vi "Plotter_UI_Event_Handler.vi"(8 "error in (no error)":errorcluster, 11 "Globals":T1) -> (0 "error out":errorcluster)   [LabVIEW 2017]
uses:
  Controls/Plotter_Globals.ctl
  Classes/ADCP.lvclass
  Controls/Plotter_Queues.ctl
  Controls/Plotter_Queue_Command_and_Data.ctl
  Controls/Plotter_Commands.ctl
  Controls/Plotter_Parameter_List_Record.ctl
panel:
  out "Send parameter":bool
  out "Exit Application":bool
  out "Enable / disable node connection":bool
  out "Remove receive parameter":bool
  out "Add receive parameter":bool
  out "Set Session Name":bool
  out "Load Symbol File":bool
  out "Serial Port Connection":bool
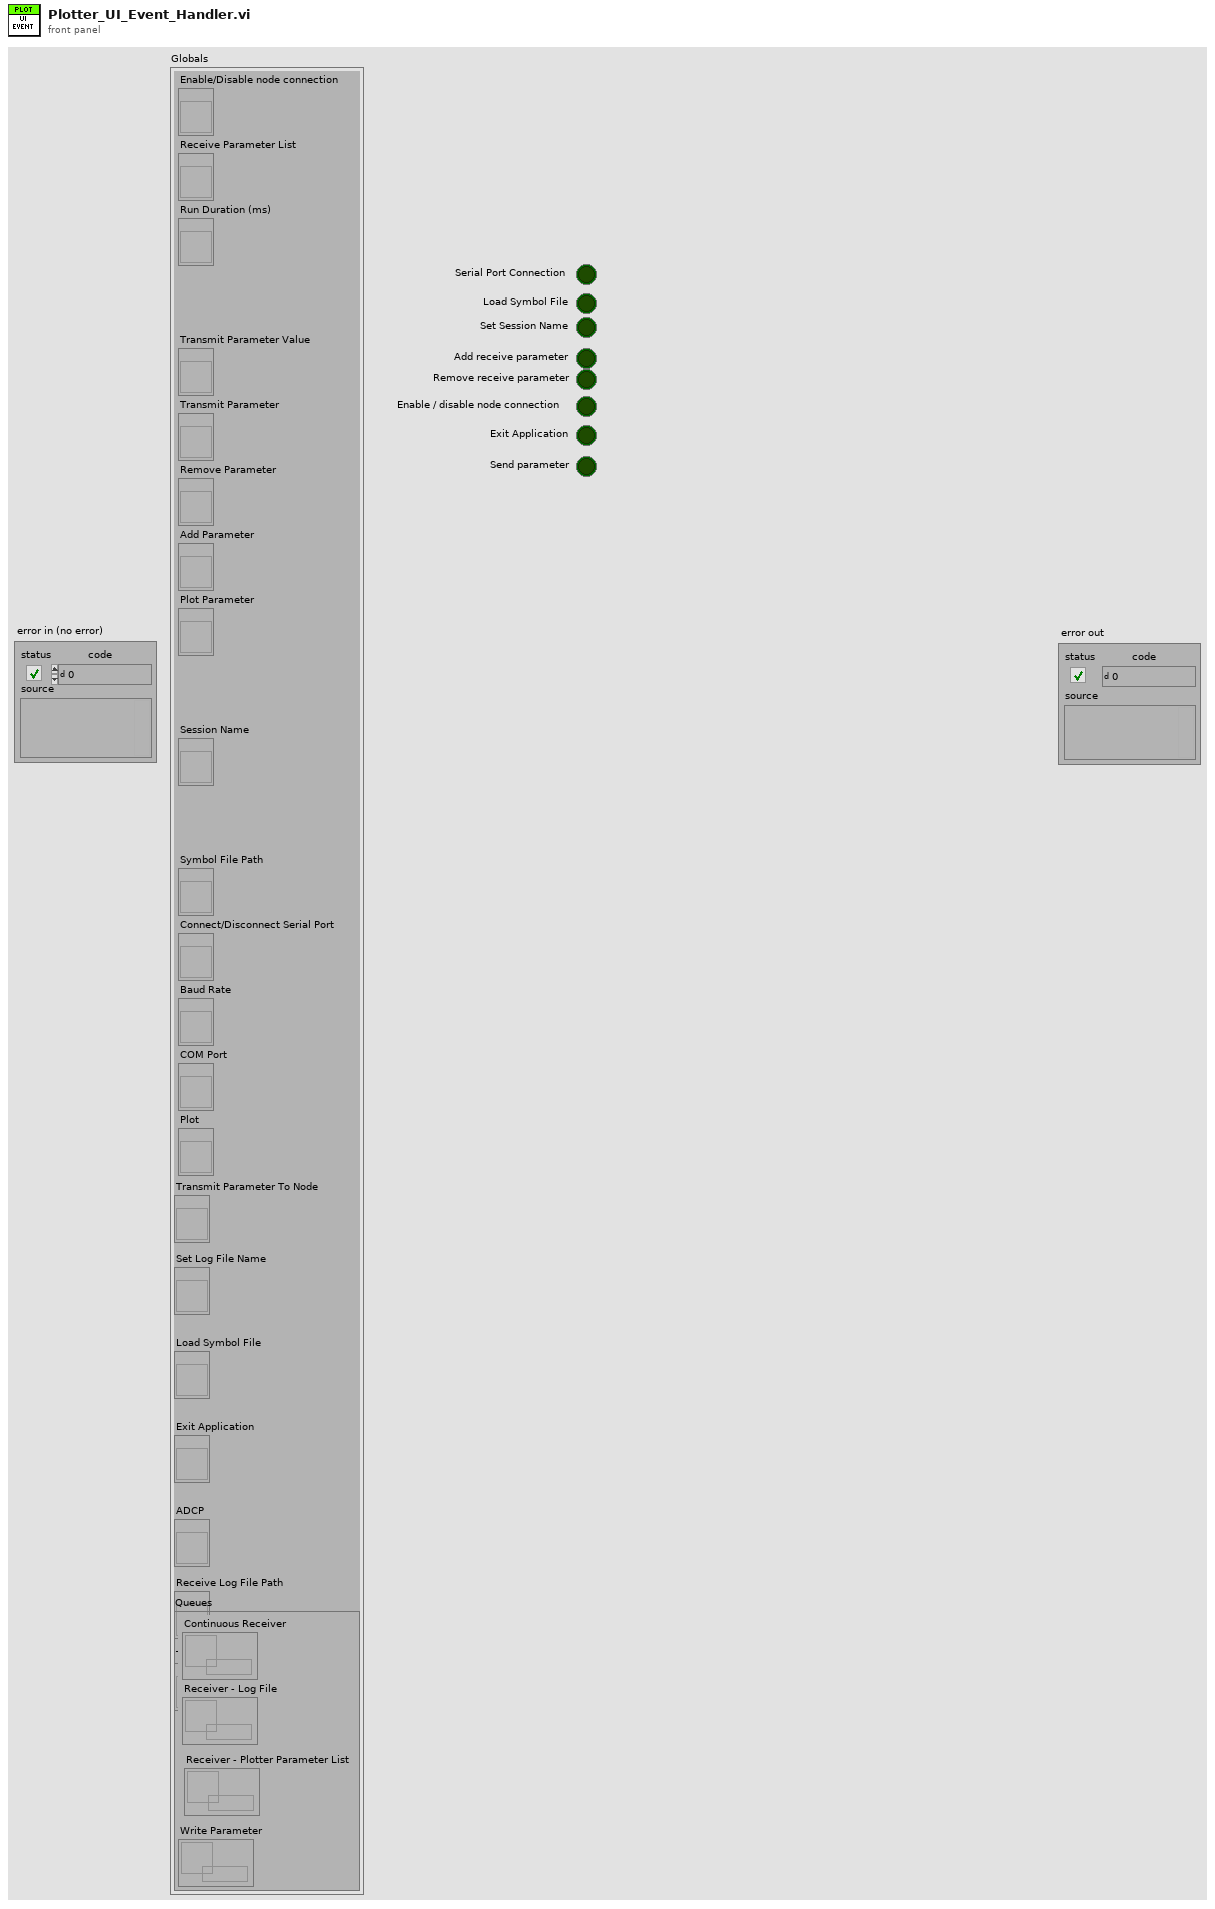
[diagram p1: front panel]
types:
  T1 = typedef "Plotter_Globals.ctl" = cluster{"Enable/Disable node connection":refnum<vi>, "Receive Parameter List":refnum<vi>, "Run Duration (ms)":refnum<vi>, "Transmit Parameter Value":refnum<vi>, "Transmit Parameter":refnum<vi>, "Remove Parameter":refnum<vi>, "Add Parameter":refnum<vi>, "Plot Parameter":refnum<vi>, "Session Name":refnum<vi>, "Symbol File Path":refnum<vi>, "Connect/Disconnect Serial Port":refnum<vi>, "Baud Rate":refnum<vi>, "COM Port":refnum<vi>, "Plot":refnum<vi>, "Transmit Parameter To Node":refnum<vi>, "Set Log File Name":refnum<vi>, "Load Symbol File":refnum<vi>, "Exit Application":refnum<vi>, "ADCP":refnum<vi>, "Transmit Log File Path":refnum<vi>, "Receive Log File Path":refnum<vi>, "Queues":T2}
  T2 = typedef "Plotter_Queues.ctl" = cluster{"Continuous Receiver":refnum<queue>, "Receiver - Log File":refnum<queue>, "Receiver - Plotter Parameter List":refnum<queue>, "Write Parameter":refnum<queue>}
  T3 = typedef "Plotter_Queue_Command_and_Data.ctl" = cluster{"Commands":T4, "Data":variant}
  T4 = typedef "Plotter_Commands.ctl" = enum16{"Idle", "Cont_RX_Open_Node", "Cont_RX_Flush_Serial_Port", "Cont_Rx_Log_Write", "Plot_Update", "Exit"}
  T5 = cluster{"Symbol File Path":path, "Transmit Log File Path":path, "Receive Log File Path":path, "COM Port":refnum<visa-resource-name>, "Baud rate":u32, "Number of retries":u16, "Retry interval (ms)":u16, "Session start time (ms)":u32, "Current time (ms)":u32, "Serialport timeout (ms)":u32}
  T6 = typedef "Plotter_Parameter_List_Record.ctl" = cluster{"Parameter":string, "Value":string}
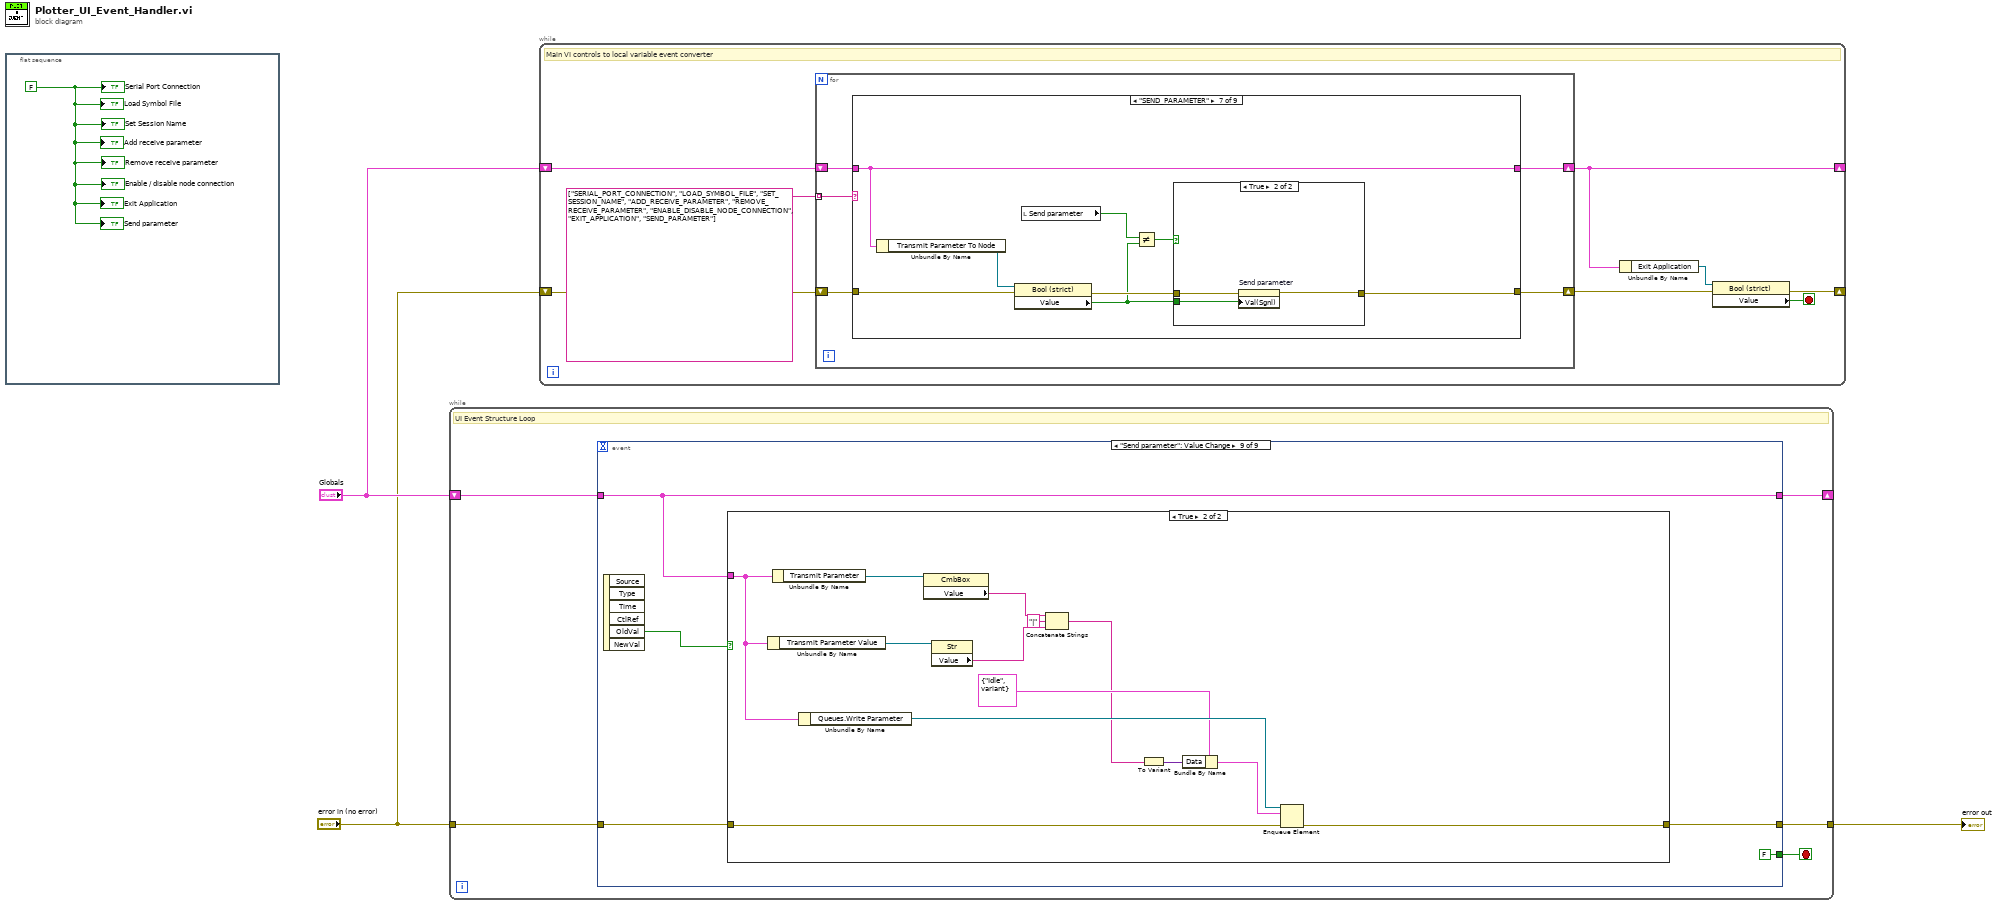
[diagram p0: block diagram]
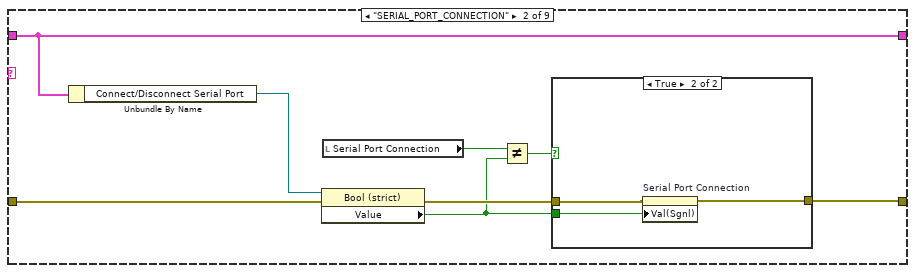
[diagram p3: hidden frame]
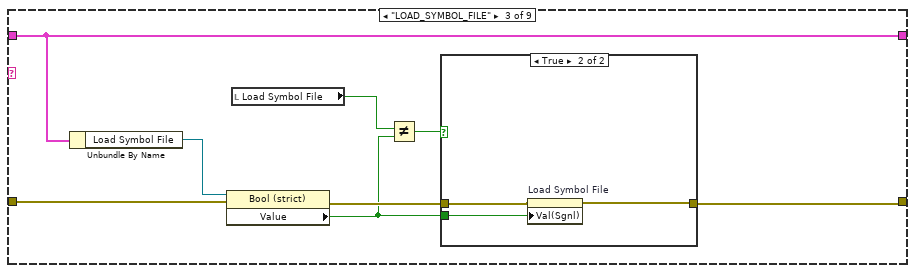
[diagram p5: hidden frame]
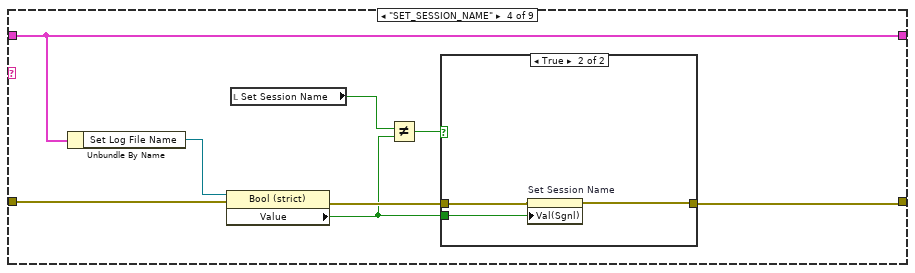
[diagram p7: hidden frame]
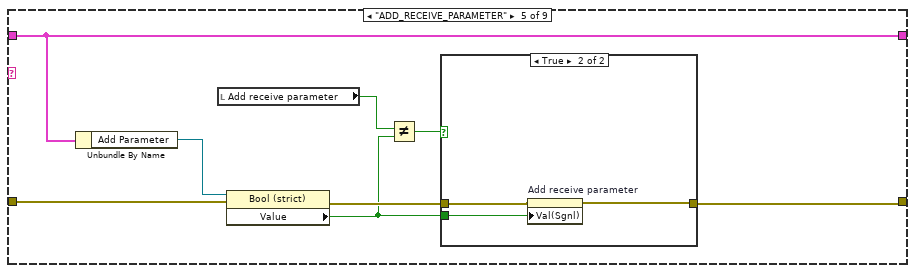
[diagram p9: hidden frame]
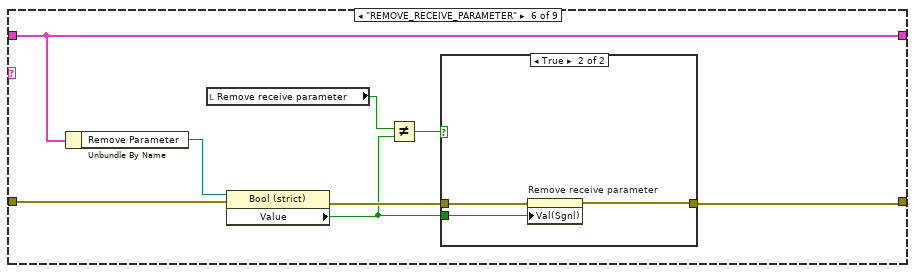
[diagram p11: hidden frame]
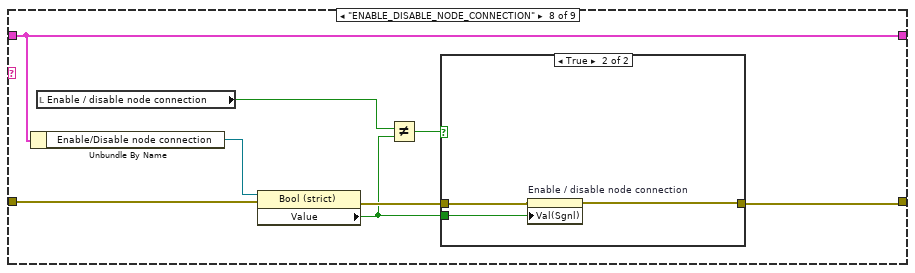
[diagram p14: hidden frame]
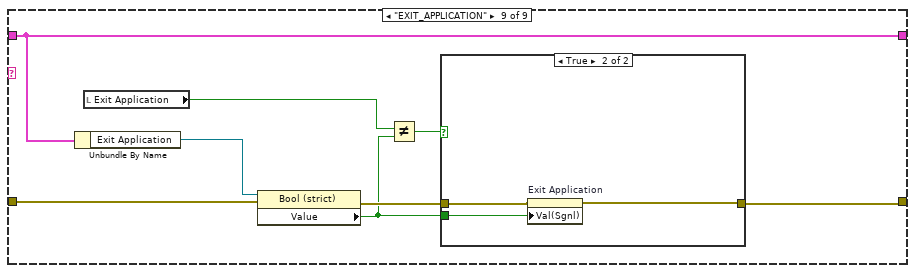
[diagram p16: hidden frame]
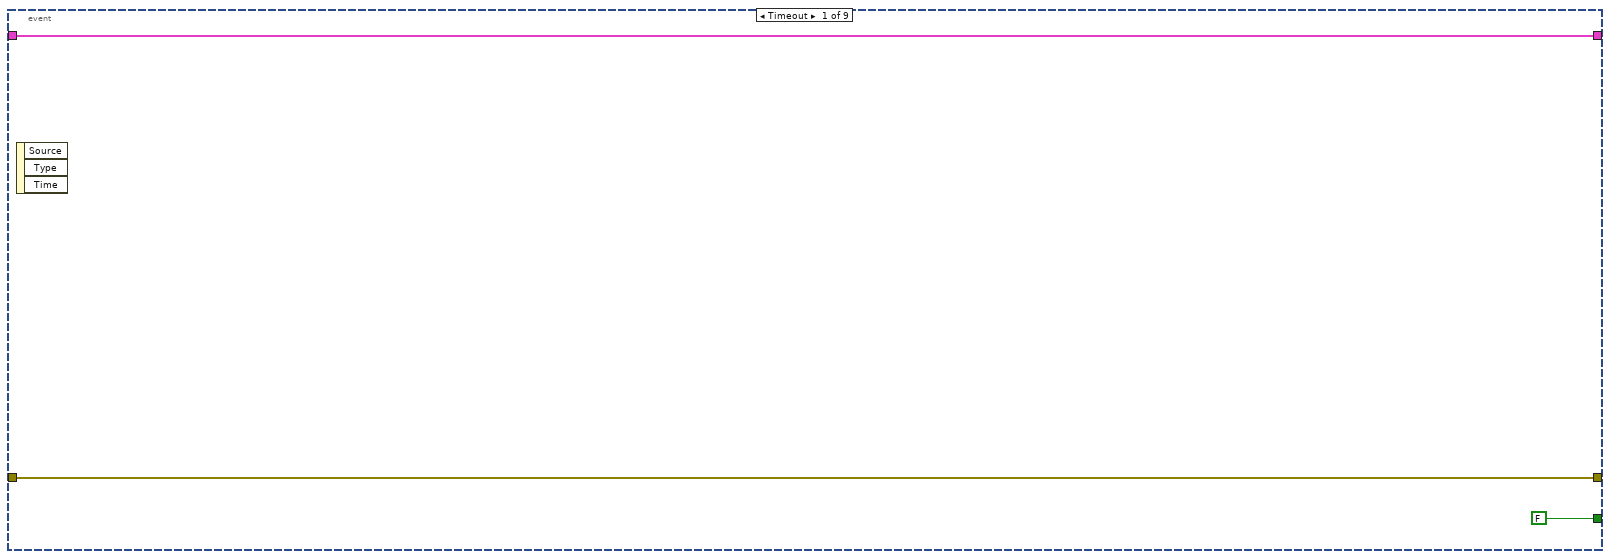
[diagram p18: hidden frame]
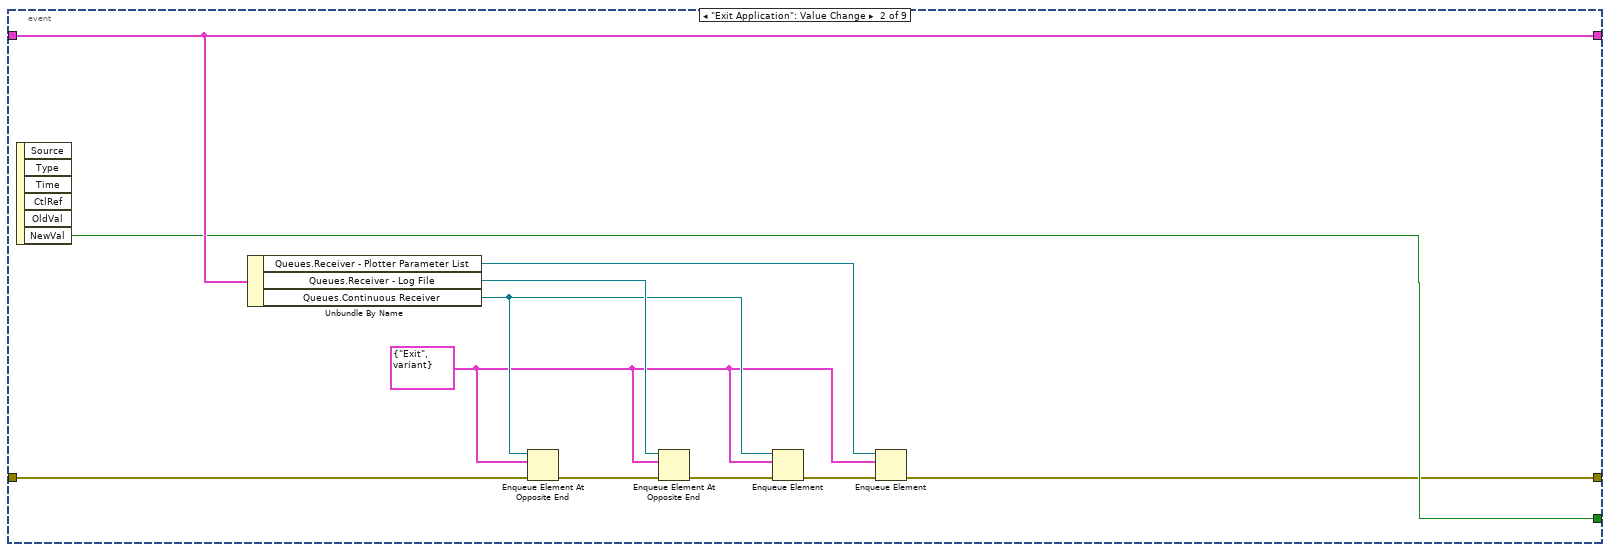
[diagram p19: hidden frame]
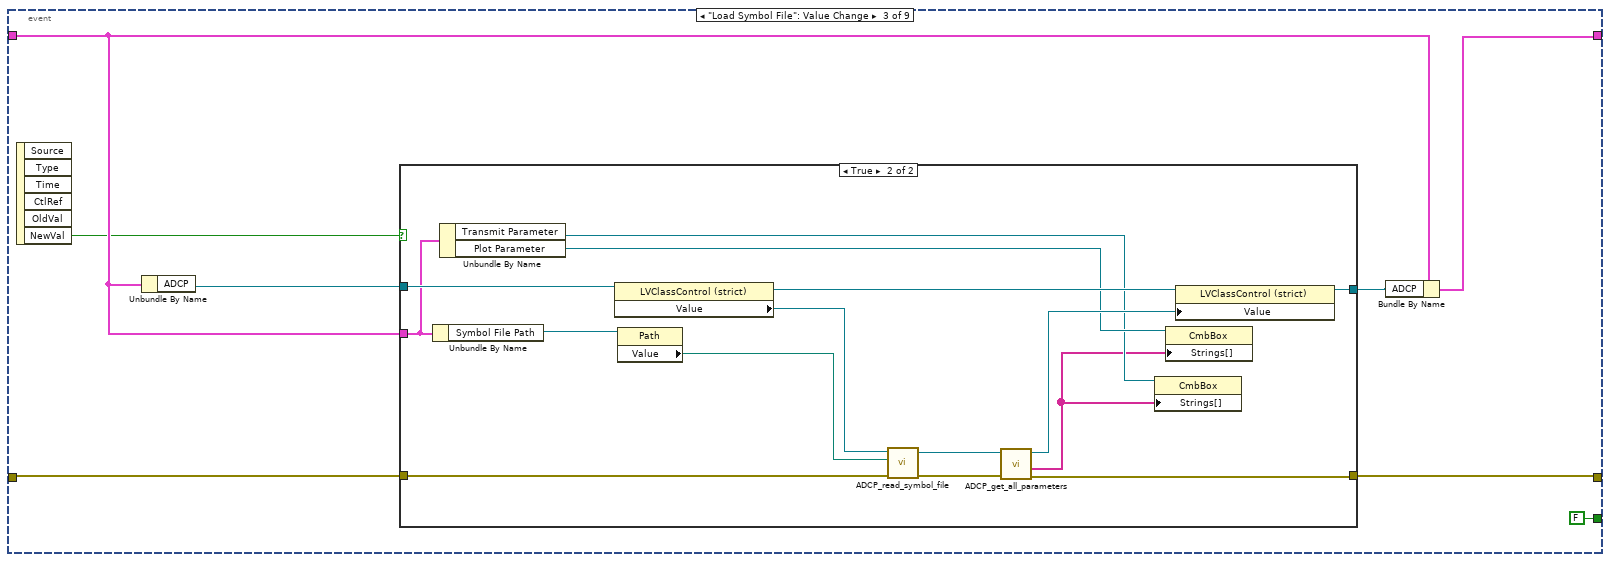
[diagram p20: hidden frame]
diagram:
  n1 = flat-sequence {
    frame #0 {
      w4 = FALSE ("Serial Port Connection")
      "Serial Port Connection" <- w4
      "Load Symbol File" <- w4
      "Set Session Name" <- w4
      "Add receive parameter" <- w4
      "Remove receive parameter" <- w4
      "Enable / disable node connection" <- w4
      "Exit Application" <- w4
      "Send parameter" <- w4
    }
  }
  n2 = while {
    shift-right: [w8] -> _
    shift-left: "Globals" -> [w9]
    tunnel: "error in (no error)" -> [w6]
    tunnel: [w5] -> w3
    stop <- w7 stop-if-true
    # "UI Event Structure Loop"
    n3 = event shown="[8] \"Send parameter\": Value Change" {
      selector: _ -> [_ _ _ _ _ _ _ _ _]
      dyn-events: _ -> [_ _ _ _ _ _ _ _ _]
      timeout: _ -> [_ _ _ _ _ _ _ _ _]
      tunnel: w9 -> [w12 w23 w27 w50 w68 w105 w130 w156 w175]
      tunnel: [w12 w23 w25 w49 w67 w103 w129 w155 w175] -> w8
      tunnel: [FALSE w17 FALSE FALSE FALSE FALSE FALSE ("NewVal") FALSE ("NewVal") FALSE ("NewVal")] -> w7
      tunnel: w6 -> [w10 w22 w31 w52 w69 w101 w131 w157 w177]
      tunnel: [w10 w15 w28 w51 w66 w100 w127 w153 w176] -> w5
      event Timeout {
        n4 = event-data() -> ()  [unwired: 1 in, 3 out]
      }
      event "Exit Application": Value Change {
        w13 = T3 {"Commands"=enum."Exit", "Data"=variant} ("element")
        n5 = event-data() -> ("NewVal"=w17:bool)  [unwired: 1 in, 5 out]
        n6 = Unbundle By Name(w23) -> ("Queues.Receiver - Plotter Parameter List"=w14:refnum<queue>, "Queues.Receiver - Log File"=w20:refnum<queue>, "Queues.Continuous Receiver"=w18:refnum<queue>)
        n7 = Enqueue Element At Opposite End(queue=w18, element=w13, error in (no error)=w22) -> (error out=w21:errorcluster)  [unwired: 1 in, 2 out]
        n8 = Enqueue Element At Opposite End(queue=w20, element=w13, error in (no error)=w21) -> (error out=w19:errorcluster)  [unwired: 1 in, 2 out]
        n9 = Enqueue Element(queue=w18, element=w13, error in (no error)=w19) -> (error out=w16:errorcluster)  [unwired: 1 in, 2 out]
        n10 = Enqueue Element(queue=w14, element=w13, error in (no error)=w16) -> (error out=w15:errorcluster)  [unwired: 1 in, 2 out]
      }
      event "Load Symbol File": Value Change {
        n11 = event-data() -> ("NewVal"=w24:bool)  [unwired: 1 in, 5 out]
        n12 = Unbundle By Name(w27) -> ("ADCP"=w30:refnum<vi>)
        n13 = case shown="True" w24 {
          tunnel: w31 -> [w32 w48]
          tunnel: w30 -> [w33 w47]
          tunnel: [w32 w40] -> w28
          tunnel: w27 -> [_ w37]
          tunnel: [w33 w42] -> w26
          frame False {
          }
          frame True {
            n14 = Unbundle By Name(w37) -> ("Symbol File Path"=w45:refnum<vi>)
            n15 = Unbundle By Name(w37) -> ("Transmit Parameter"=w35:refnum<vi>, "Plot Parameter"=w36:refnum<vi>)
            n16 = property class="LVClassControl (strict)"(reference=w47) -> (reference out=w43:refnum<vi>, "Value"=w46:refnum<class "ADCP.lvclass">)  [unwired: 1 in, 1 out]
            n17 = property class="Path"(reference=w45) -> ("Value"=w44:path)  [unwired: 1 in, 2 out]
            n18 = call "ADCP_read_symbol_file.vi"("error in (no error)"=w48, "Symbol File Path"=w44, "ADCP in"=w46) -> ("error out"=w41:errorcluster, "ADCP out"=w39:refnum<class "ADCP.lvclass">)  [unwired: 5 in, 2 out]
            n19 = call "ADCP_get_all_parameters.vi"("error in (no error)"=w41, "ADCP In"=w39) -> ("error out"=w40:errorcluster, "Parameter names"=w34:string[], "ADCP Out"=w38:refnum<class "ADCP.lvclass">)  [unwired: 6 in, 1 out]
            n20 = property class="CmbBox"(reference=w35, "Strings[]"=w34) -> ()  [unwired: 1 in, 2 out]
            n21 = property class="CmbBox"(reference=w36, "Strings[]"=w34) -> ()  [unwired: 1 in, 2 out]
            n22 = property class="LVClassControl (strict)"(reference=w43, "Value"=w38) -> (reference out=w42:refnum<vi>)  [unwired: 1 in, 1 out]
          }
        }
        n23 = Bundle By Name(cluster=w27, "ADCP"=w26) -> (w25:T1)
      }
      event "Set Session Name": Value Change {
        n24 = event-data() -> ("NewVal"=w53:bool)  [unwired: 1 in, 5 out]
        n25 = case shown="True" w53 {
          tunnel: w52 -> [w56 w64]
          tunnel: [w56 w60] -> w51
          tunnel: w50 -> [w55 w59]
          tunnel: [w55 w59] -> w49
          frame False {
          }
          frame True {
            n26 = Unbundle By Name(w59) -> ("Session Name"=w58:refnum<vi>)
            n27 = property class="Str"(reference=w58) -> ("Value"=w57:string)  [unwired: 1 in, 2 out]
            n28 = call "Transmit_Log_File_FGV.vi"("Session name"=w57, "error in (no error)"=w64, "Command"=enum16{"Initialize", "Update", "Stop"}."Initialize") -> ("error out"=w62:errorcluster)  [unwired: 7 in, 1 out]
            n29 = call "Receive_Log_File_FGV.vi"("Session name"=w57, "error in (no error)"=w62, "Command"=enum16{"Initialize", "Update", "Stop"}."Initialize") -> ("error out"=w60:errorcluster)  [unwired: 7 in, 1 out]
          }
        }
      }
      event "Enable / disable node connection": Value Change {
        n30 = event-data() -> ("NewVal"=w70:bool)  [unwired: 1 in, 5 out]
        n31 = case shown="False" w70 {
          tunnel: w69 -> [w82 w92]
          tunnel: w68 -> [w71 w91]
          tunnel: [w76 w95] -> w67
          tunnel: [w72 w88] -> w66
          frame True {
            n32 = Unbundle By Name(w71) -> ("ADCP"=w83:refnum<vi>)
            n33 = property class="LVClassControl (strict)"(reference=w83) -> (reference out=w80:refnum<vi>, error out=w79:errorcluster, "Value"=w81:refnum<class "ADCP.lvclass">)  [unwired: 1 in]
            n34 = call "ADCP_Open_Node_Connection.vi"("error in (no error)"=w82, "ADCP In"=w81) -> ("error out"=w73:errorcluster, "ADCP Out"=w78:refnum<class "ADCP.lvclass">)  [unwired: 8 in]
            n35 = property class="LVClassControl (strict)"(reference=w80, error in=w79, "Value"=w78) -> (reference out=w77:refnum<vi>)  [unwired: 1 out]
            n36 = Unbundle By Name(w71) -> ("Queues.Continuous Receiver"=w75:refnum<queue>)
            n37 = Bundle By Name(cluster=w71, "ADCP"=w77) -> (w76:T1)
            n38 = Enqueue Element(queue=w75, element=T3 {"Commands"=enum."Cont_RX_Open_Node", "Data"=variant}, error in (no error)=w73) -> (error out=w72:errorcluster)  [unwired: 1 in, 2 out]
          }
          frame False {
            n39 = Unbundle By Name(w91) -> ("Queues.Continuous Receiver"=w87:refnum<queue>)
            n40 = Unbundle By Name(w91) -> ("ADCP"=w99:refnum<vi>)
            n41 = property class="LVClassControl (strict)"(reference=w99) -> (reference out=w98:refnum<vi>, error out=w97:errorcluster, "Value"=w94:refnum<class "ADCP.lvclass">)  [unwired: 1 in]
            n42 = call "ADCP_Close_Node_Connection.vi"("error in (no error)"=w92, "ADCP In"=w94) -> ("error out"=w90:errorcluster, "ADCP Out"=w93:refnum<class "ADCP.lvclass">)  [unwired: 8 in]
            n43 = property class="LVClassControl (strict)"(reference=w98, error in=w97, "Value"=w93) -> (reference out=w96:refnum<vi>)  [unwired: 1 out]
            n44 = Enqueue Element(queue=w87, element=T3 {"Commands"=enum."Cont_RX_Flush_Serial_Port", "Data"=variant}, error in (no error)=w90) -> (queue out=w86:refnum<queue>, error out=w89:errorcluster)  [unwired: 1 in, 1 out]
            n45 = Enqueue Element(queue=w86, element=T3 {"Commands"=enum."Idle", "Data"=variant}, error in (no error)=w89) -> (error out=w88:errorcluster)  [unwired: 1 in, 2 out]
            n46 = Bundle By Name(cluster=w91, "ADCP"=w96) -> (w95:T1)
          }
        }
      }
      event "Serial Port Connection": Value Change {
        n47 = event-data() -> ("NewVal"=w104:bool)  [unwired: 1 in, 5 out]
        n48 = case shown="True" w104 {
          tunnel: w105 -> [w107 w109]
          tunnel: [w107 w120] -> w103
          tunnel: w101 -> [w106 w125]
          tunnel: [w106 w108] -> w100
          frame False {
          }
          frame True {
            n49 = Unbundle By Name(w109) -> ("COM Port"=w118:refnum<vi>, "Baud Rate"=w116:refnum<vi>)
            n50 = Unbundle By Name(w109) -> ("ADCP"=w126:refnum<vi>)
            n51 = property class="LVClassControl (strict)"(reference=w126) -> (reference out=w123:refnum<vi>, "Value"=w124:refnum<class "ADCP.lvclass">)  [unwired: 1 in, 1 out]
            n52 = property class="DigNum (strict)"(reference=w116) -> ("Value"=w115:u32)  [unwired: 1 in, 2 out]
            n53 = property class="VISAName"(reference=w118) -> ("Value"=w117:refnum<visa-resource-name>)  [unwired: 1 in, 2 out]
            n54 = Tick Count (ms)() -> (millisecond timer value=w111:u32)
            n55 = Bundle By Name(cluster=T5 {"Symbol File Path"=path "", "Transmit Log File Path"=path "", "Receive Log File Path"=path "", "COM Port"="", "Baud rate"=0, "Number of retries"=0, "Retry interval (ms)"=0, "Session start time (ms)"=0, "Current time (ms)"=0, "Serialport timeout (ms)"=0} ("ADCP Session Parameters"), "COM Port"=w117, "Baud rate"=w115, "Number of retries"=u16 10, "Retry interval (ms)"=u16 250, "Session start time (ms)"=w111, "Serialport timeout (ms)"=u32 1000) -> (w114:T5)
            n56 = call "ADCP_Init_Session.vi"("error in (no error)"=w125, "ADCP Session Parameters"=w114, "ADCP in"=w124) -> ("error out"=w108:errorcluster, "ADCP out"=w122:refnum<class "ADCP.lvclass">)  [unwired: 7 in]
            n57 = property class="LVClassControl (strict)"(reference=w123, "Value"=w122) -> (reference out=w121:refnum<vi>)  [unwired: 1 in, 1 out]
            n58 = Bundle By Name(cluster=w109, "ADCP"=w121) -> (w120:T1)
          }
        }
      }
      event "Add receive parameter": Value Change {
        n59 = event-data() -> ("NewVal"=w132:bool)  [unwired: 1 in, 5 out]
        n60 = case shown="True" w132 {
          tunnel: w131 -> [w133 w137]
          tunnel: w130 -> [w134 w143]
          tunnel: [w134 w143] -> w129
          tunnel: [w133 w137] -> w127
          frame False {
          }
          frame True {
            n61 = Unbundle By Name(w143) -> ("Receive Parameter List"=w142:refnum<vi>)
            n62 = Unbundle By Name(w143) -> ("Plot Parameter"=w144:refnum<vi>)
            n63 = property class="Arr (strict)"(reference=w142) -> (reference out=w139:refnum<vi>, "Value"=w140:T6[])  [unwired: 1 in, 1 out]
            n64 = property class="CmbBox"(reference=w144) -> ("Value"=w135:string)  [unwired: 1 in, 2 out]
            n65 = for {
              tunnel: w140 -> [w152] mode=indexing
              tunnel: [w151] -> w141 mode=indexing
              n66 = Unbundle By Name(w152) -> ("Parameter"=w151:string)
            }
            n67 = Search 1D Array(1D array=w141, element=w135) -> (index of element=w136:i32)  [unwired: 1 in]
            n68 = case shown="-1" w136 {
              tunnel: w140 -> [w145 w150]
              tunnel: [w145 w149] -> w138
              tunnel: w135 -> [_ w148]
              frame 0, Default {
              }
              frame -1 {
                n69 = Bundle By Name(cluster=T6 {"Parameter"="", "Value"=""} ("Cluster"), "Parameter"=w148) -> (w146:T6)
                n70 = Build Array (concatenate)(w150, w146) -> (w149:T6[])
              }
            }
            n71 = property class="Arr (strict)"(reference=w139, "Value"=w138) -> ()  [unwired: 1 in, 2 out]
          }
        }
      }
      event "Remove receive parameter": Value Change {
        n72 = event-data() -> ("NewVal"=w158:bool)  [unwired: 1 in, 5 out]
        n73 = case shown="True" w158 {
          tunnel: w157 -> [w159 w165]
          tunnel: w156 -> [w160 w170]
          tunnel: [w160 w170] -> w155
          tunnel: [w159 w165] -> w153
          frame False {
          }
          frame True {
            n74 = Unbundle By Name(w170) -> ("Receive Parameter List"=w169:refnum<vi>)
            n75 = Unbundle By Name(w170) -> ("Plot Parameter"=w171:refnum<vi>)
            n76 = property class="Arr (strict)"(reference=w169) -> (reference out=w166:refnum<vi>, "Value"=w164:T6[])  [unwired: 1 in, 1 out]
            n77 = property class="CmbBox"(reference=w171) -> ("Value"=w167:string)  [unwired: 1 in, 2 out]
            n78 = for {
              tunnel: w164 -> [w173] mode=indexing
              tunnel: [w172] -> w168 mode=indexing
              n79 = Unbundle By Name(w173) -> ("Parameter"=w172:string)
            }
            n80 = Search 1D Array(1D array=w168, element=w167) -> (index of element=w161:i32)  [unwired: 1 in]
            n81 = Delete From Array(array=w164, length=1, index=w161) -> (array with subset deleted=w163:T6[])  [unwired: 1 out]
            n82 = property class="Arr (strict)"(reference=w166, "Value"=w163) -> ()  [unwired: 1 in, 2 out]
          }
        }
      }
      event "Send parameter": Value Change {
        n83 = event-data() -> ("OldVal"=w174:bool)  [unwired: 1 in, 5 out]
        n84 = case shown="True" w174 {
          tunnel: w177 -> [w179 w186]
          tunnel: [w179 w181] -> w176
          tunnel: w175 -> [_ w187]
          frame False {
          }
          frame True {
            n85 = Unbundle By Name(w187) -> ("Transmit Parameter Value"=w191:refnum<vi>)
            n86 = Unbundle By Name(w187) -> ("Transmit Parameter"=w192:refnum<vi>)
            n87 = Unbundle By Name(w187) -> ("Queues.Write Parameter"=w185:refnum<queue>)
            n88 = property class="CmbBox"(reference=w192) -> ("Value"=w189:string)  [unwired: 1 in, 2 out]
            n89 = property class="Str"(reference=w191) -> ("Value"=w190:string)  [unwired: 1 in, 2 out]
            n90 = Concatenate Strings(w189, "|" ("string"), w190) -> (w182:string)
            n91 = To Variant(anything=w182) -> (Variant=w183:variant)
            n92 = Bundle By Name(cluster=T3 {"Commands"=enum."Idle", "Data"=variant} ("element"), "Data"=w183) -> (w180:T3)
            n93 = Enqueue Element(queue=w185, element=w180, error in (no error)=w186) -> (error out=w181:errorcluster)  [unwired: 1 in, 2 out]
          }
        }
      }
    }
  }
  "error out" <- w3
  n94 = while {
    shift-right: [w193] -> _
    shift-left: "Globals" -> [w200]
    shift-right: [w194] -> _
    shift-left: "error in (no error)" -> [w198]
    stop <- w195 stop-if-true
    # "Main VI controls to local variable event converter"
    n95 = for {
      tunnel: string[] ["SERIAL_PORT_CONNECTION", "LOAD_SYMBOL_FILE", "SET_SESSION_NAME", "ADD_RECEIVE_PARAMETER", "REMOVE_RECEIVE_PARAMETER", "ENABLE_DISABLE_NODE_CONNECTION", "EXIT_APPLICATION", "SEND_PARAMETER"] -> [w205] mode=indexing
      shift-right: [w203] -> w197
      shift-left: w198 -> [w204]
      shift-right: [w201] -> w193
      shift-left: w200 -> [w202]
      n96 = case shown="\"SEND_PARAMETER\"" w205 {
        tunnel: w204 -> [w207 w215 w226 w238 w250 w262 w274 w286 w298]
        tunnel: [w207 w208 w222 w234 w246 w258 w270 w282 w294] -> w203
        tunnel: w202 -> [w206 w214 w221 w233 w245 w257 w269 w281 w293]
        tunnel: [w206 w214 w221 w233 w245 w257 w269 w281 w293] -> w201
        frame Default {
        }
        frame "SERIAL_PORT_CONNECTION" {
          n97 = Unbundle By Name(w214) -> ("Connect/Disconnect Serial Port"=w213:refnum<vi>)
          n98 = property class="Bool (strict)"(reference=w213, error in=w215) -> (error out=w210:errorcluster, "Value"=w209:bool)  [unwired: 1 out]
          n99 = local read "Serial Port Connection"() -> (w212:bool)
          n100 = Not Equal?(x=w212, y=w209) -> (x != y?=w211:bool)
          n101 = case shown="True" w211 {
            tunnel: w210 -> [w216 w219]
            tunnel: w209 -> [_ w218]
            tunnel: [w216 w217] -> w208
            frame False {
            }
            frame True {
              n102 = property on="Serial Port Connection" class="Bool (strict)"(error in=w219, "Val(Sgnl)"=w218) -> (error out=w217:errorcluster)  [unwired: 1 in, 1 out]
            }
          }
        }
        frame "LOAD_SYMBOL_FILE" {
          n103 = Unbundle By Name(w221) -> ("Load Symbol File"=w227:refnum<vi>)
          n104 = property class="Bool (strict)"(reference=w227, error in=w226) -> (error out=w223:errorcluster, "Value"=w220:bool)  [unwired: 1 out]
          n105 = local read "Load Symbol File"() -> (w225:bool)
          n106 = Not Equal?(x=w225, y=w220) -> (x != y?=w224:bool)
          n107 = case shown="True" w224 {
            tunnel: w223 -> [w228 w231]
            tunnel: [w228 w230] -> w222
            tunnel: w220 -> [_ w229]
            frame False {
            }
            frame True {
              n108 = property on="Load Symbol File" class="Bool (strict)"(error in=w231, "Val(Sgnl)"=w229) -> (error out=w230:errorcluster)  [unwired: 1 in, 1 out]
            }
          }
        }
        frame "SET_SESSION_NAME" {
          n109 = Unbundle By Name(w233) -> ("Set Log File Name"=w239:refnum<vi>)
          n110 = property class="Bool (strict)"(reference=w239, error in=w238) -> (error out=w235:errorcluster, "Value"=w232:bool)  [unwired: 1 out]
          n111 = local read "Set Session Name"() -> (w237:bool)
          n112 = Not Equal?(x=w237, y=w232) -> (x != y?=w236:bool)
          n113 = case shown="True" w236 {
            tunnel: w235 -> [w240 w243]
            tunnel: [w240 w242] -> w234
            tunnel: w232 -> [_ w241]
            frame False {
            }
            frame True {
              n114 = property on="Set Session Name" class="Bool (strict)"(error in=w243, "Val(Sgnl)"=w241) -> (error out=w242:errorcluster)  [unwired: 1 in, 1 out]
            }
          }
        }
        frame "ADD_RECEIVE_PARAMETER" {
          n115 = Unbundle By Name(w245) -> ("Add Parameter"=w251:refnum<vi>)
          n116 = local read "Add receive parameter"() -> (w249:bool)
          n117 = property class="Bool (strict)"(reference=w251, error in=w250) -> (error out=w247:errorcluster, "Value"=w244:bool)  [unwired: 1 out]
          n118 = Not Equal?(x=w249, y=w244) -> (x != y?=w248:bool)
          n119 = case shown="True" w248 {
            tunnel: w247 -> [w252 w255]
            tunnel: [w252 w254] -> w246
            tunnel: w244 -> [_ w253]
            frame False {
            }
            frame True {
              n120 = property on="Add receive parameter" class="Bool (strict)"(error in=w255, "Val(Sgnl)"=w253) -> (error out=w254:errorcluster)  [unwired: 1 in, 1 out]
            }
          }
        }
        frame "REMOVE_RECEIVE_PARAMETER" {
          n121 = Unbundle By Name(w257) -> ("Remove Parameter"=w263:refnum<vi>)
          n122 = local read "Remove receive parameter"() -> (w261:bool)
          n123 = property class="Bool (strict)"(reference=w263, error in=w262) -> (error out=w259:errorcluster, "Value"=w256:bool)  [unwired: 1 out]
          n124 = Not Equal?(x=w261, y=w256) -> (x != y?=w260:bool)
          n125 = case shown="True" w260 {
            tunnel: w259 -> [w264 w267]
            tunnel: [w264 w266] -> w258
            tunnel: w256 -> [_ w265]
            frame False {
            }
            frame True {
              n126 = property on="Remove receive parameter" class="Bool (strict)"(error in=w267, "Val(Sgnl)"=w265) -> (error out=w266:errorcluster)  [unwired: 1 in, 1 out]
            }
          }
        }
        frame "SEND_PARAMETER" {
          n127 = Unbundle By Name(w269) -> ("Transmit Parameter To Node"=w275:refnum<vi>)
          n128 = property class="Bool (strict)"(reference=w275, error in=w274) -> (error out=w271:errorcluster, "Value"=w268:bool)  [unwired: 1 out]
          n129 = local read "Send parameter"() -> (w273:bool)
          n130 = Not Equal?(x=w273, y=w268) -> (x != y?=w272:bool)
          n131 = case shown="True" w272 {
            tunnel: w271 -> [w276 w279]
            tunnel: [w276 w278] -> w270
            tunnel: w268 -> [_ w277]
            frame False {
            }
            frame True {
              n132 = property on="Send parameter" class="Bool (strict)"(error in=w279, "Val(Sgnl)"=w277) -> (error out=w278:errorcluster)  [unwired: 1 in, 1 out]
            }
          }
        }
        frame "ENABLE_DISABLE_NODE_CONNECTION" {
          n133 = Unbundle By Name(w281) -> ("Enable/Disable node connection"=w287:refnum<vi>)
          n134 = local read "Enable / disable node connection"() -> (w285:bool)
          n135 = property class="Bool (strict)"(reference=w287, error in=w286) -> (error out=w283:errorcluster, "Value"=w280:bool)  [unwired: 1 out]
          n136 = Not Equal?(x=w285, y=w280) -> (x != y?=w284:bool)
          n137 = case shown="True" w284 {
            tunnel: w283 -> [w288 w291]
            tunnel: [w288 w290] -> w282
            tunnel: w280 -> [_ w289]
            frame False {
            }
            frame True {
              n138 = property on="Enable / disable node connection" class="Bool (strict)"(error in=w291, "Val(Sgnl)"=w289) -> (error out=w290:errorcluster)  [unwired: 1 in, 1 out]
            }
          }
        }
        frame "EXIT_APPLICATION" {
          n139 = Unbundle By Name(w293) -> ("Exit Application"=w299:refnum<vi>)
          n140 = local read "Exit Application"() -> (w297:bool)
          n141 = property class="Bool (strict)"(reference=w299, error in=w298) -> (error out=w295:errorcluster, "Value"=w292:bool)  [unwired: 1 out]
          n142 = Not Equal?(x=w297, y=w292) -> (x != y?=w296:bool)
          n143 = case shown="True" w296 {
            tunnel: w295 -> [w300 w303]
            tunnel: [w300 w302] -> w294
            tunnel: w292 -> [_ w301]
            frame False {
            }
            frame True {
              n144 = property on="Exit Application" class="Bool (strict)"(error in=w303, "Val(Sgnl)"=w301) -> (error out=w302:errorcluster)  [unwired: 1 in, 1 out]
            }
          }
        }
      }
    }
    n145 = Unbundle By Name(w193) -> ("Exit Application"=w196:refnum<vi>)
    n146 = property class="Bool (strict)"(reference=w196, error in=w197) -> (error out=w194:errorcluster, "Value"=w195:bool)  [unwired: 1 out]
  }
